vi "Motor.vi"(7 "Motor Input":dbl, 8 "error in (no error)":errorcluster, 9 "Victor SPX?":bool, 10 "Refnum Name":string="My Motor RefNum", 11 "Device Number":u8) -> (0 "error out":errorcluster)   [LabVIEW 2018]
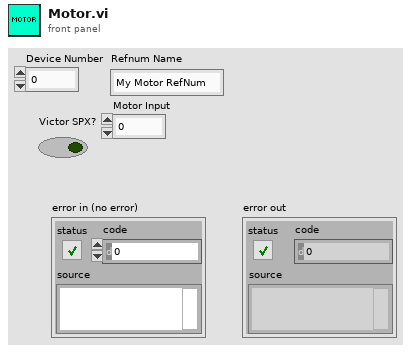
[diagram p1: front panel]
types:
  T1 = typedef "WPI_MotorControlDeviceRef.ctl" = cluster{"DeviceStatus":errorcluster, "Type":T2, "PWM":cluster{"PWM Channel":T3, "DeadBand":T4}, "CAN":cluster{"Device Number":u8, "SetOutput VI Ref":variant, "GetOutput VI Ref":variant, "Enable VI Ref":variant, "Disable VI Ref":variant, "Data":variant}, "Invert":bool, "DIO PWM":cluster{"PWM \"Enable\" Channel":T3, "DIOChannel":T5, "PWM Rate":dbl}}
  T2 = typedef "WPI_MotorControlType.ctl" = enum16{"PWM", "CAN", "DIO PWM"}
  T3 = typedef "FPGA_DIOPWMChannel.ctl" = enum8{"PWM 0", "PWM 1", "PWM 2", "PWM 3", "PWM 4", "PWM 5", "PWM 6", "PWM 7", "PWM 8", "PWM 9", "PWM MXP 0", "PWM MXP 1", "PWM MXP 2", "PWM MXP 3", "PWM MXP 4", "PWM MXP 5", "PWM MXP 6", "PWM MXP 7", "PWM MXP 8", "PWM MXP 9", "Invalid"}
  T4 = typedef "WPI_PWMDeadband.ctl" = cluster{"Name":string, "maxPositivePwm":i32, "minPositivePwm":i32, "centerPwm":i32, "maxNegativePwm":i32, "minNegativePwm":i32, "angularRange":u16}
  T5 = typedef "FPGA_DIOChannel.ctl" = enum8{"DIO 0", "DIO 1", "DIO 2", "DIO 3", "DIO 4", "DIO 5", "DIO 6", "DIO 7", "DIO 8", "DIO 9", "DIO MXP 0", "DIO MXP 1", "DIO MXP 2", "DIO MXP 3", "DIO MXP 4", "DIO MXP 5", "DIO MXP 6", "DIO MXP 7", "DIO MXP 8", "DIO MXP 9", "DIO MXP 10", "DIO MXP 11", "DIO MXP 12", "DIO MXP 13", "DIO MXP 14", "DIO MXP 15", "SPI Port CS1", "SPI Port CS2", "SPI Port CS3", "SPI Port MISO", "SPI Port MOSI", "Invalid"}
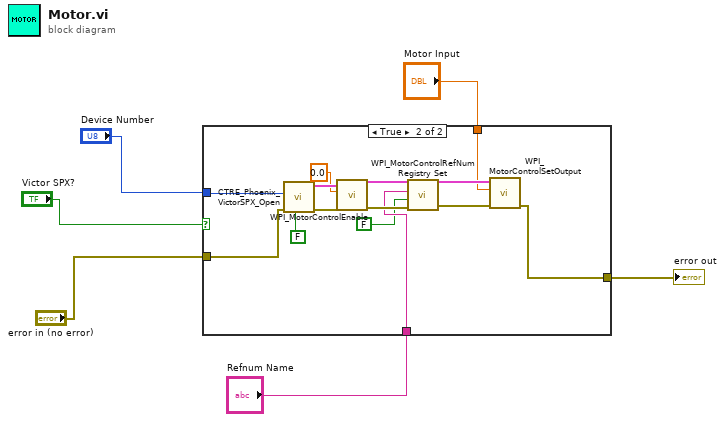
[diagram p0: block diagram]
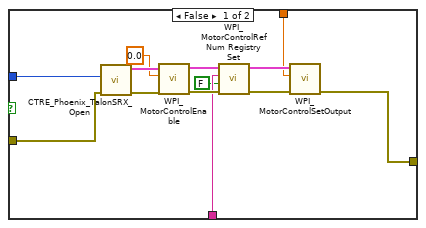
[diagram p2: hidden frame]
diagram:
  n1 = case shown="True" "Victor SPX?" {
    tunnel: "Device Number" -> [w19 w33]
    tunnel: "Refnum Name" -> [w13 w25]
    tunnel: "error in (no error)" -> [w9 w32]
    tunnel: [w8 w20] -> w2
    tunnel: "Motor Input" -> [w7 w21]
    frame False {
      n2 = call <vilib>:"CTRE_Phoenix_TalonSRX_Open.vi"("error in"=w9, "Device Number"=w19) -> ("error out"=w18:errorcluster, "CAN Talon SRX Ref"=w17:T1)  [unwired: 8 in]
      n3 = call <vilib>:"WPI_MotorControlEnable.vi"("error in (no error)"=w18, "Encoder Initial Position"=0.0, "CAN MotorDevRef"=w17) -> ("error out"=w15:errorcluster, "CAN MotorDevRef"=w14:T1)  [unwired: 7 in]
      n4 = call <vilib>:"WPI_MotorControlRefNum Registry Set.vi"("error in (no error)"=w15, "Test Mode Only"=FALSE, "refnum name"=w13, "MotorControlDevRef"=w14) -> ("error out"=w10:errorcluster, "MotorControlDevRef"=w11:T1)  [unwired: 6 in]
      n5 = call <vilib>:"WPI_MotorControlSetOutput.vi"("error in (no error)"=w10, "Output"=w7, "MotorControlDevRef"=w11) -> ("error out"=w8:errorcluster)  [unwired: 6 in, 2 out]
    }
    frame True {
      n6 = call <vilib>:"CTRE_Phoenix_VictorSPX_Open.vi"("Invert"=FALSE, "error in"=w32, "Device Number"=w33) -> ("error out"=w30:errorcluster, "CAN Talon SRX Ref"=w29:T1)  [unwired: 7 in]
      n7 = call <vilib>:"WPI_MotorControlEnable.vi"("error in (no error)"=w30, "Encoder Initial Position"=0.0, "CAN MotorDevRef"=w29) -> ("error out"=w27:errorcluster, "CAN MotorDevRef"=w26:T1)  [unwired: 7 in]
      n8 = call <vilib>:"WPI_MotorControlRefNum Registry Set.vi"("error in (no error)"=w27, "Test Mode Only"=FALSE, "refnum name"=w25, "MotorControlDevRef"=w26) -> ("error out"=w22:errorcluster, "MotorControlDevRef"=w23:T1)  [unwired: 6 in]
      n9 = call <vilib>:"WPI_MotorControlSetOutput.vi"("error in (no error)"=w22, "Output"=w21, "MotorControlDevRef"=w23) -> ("error out"=w20:errorcluster)  [unwired: 6 in, 2 out]
    }
  }
  "error out" <- w2
